vi "SR760FFT_init_measure.vi"(5 "Measure":bool, 7 "Init":bool, 8 "error in":T1, 11 "GPIB address":string="10") -> (0 "error out":T1, 3 "Array":dbl[](array[numeric]))   [LabVIEW 2023]
panel:
  out "trace":dbl[](graph)
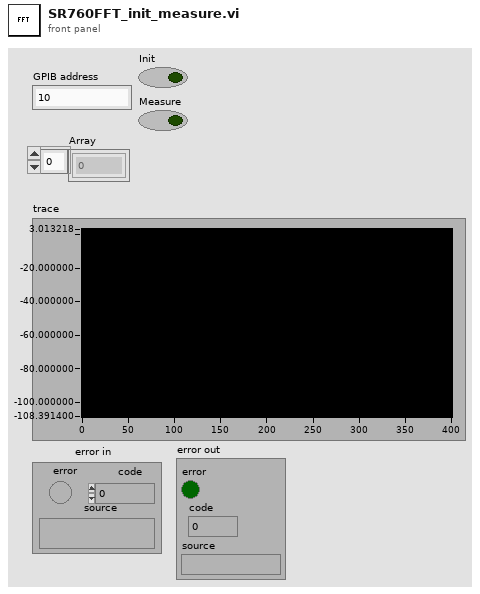
[diagram p1: front panel]
types:
  T1 = cluster{"error":bool, "code":i32, "source":string}
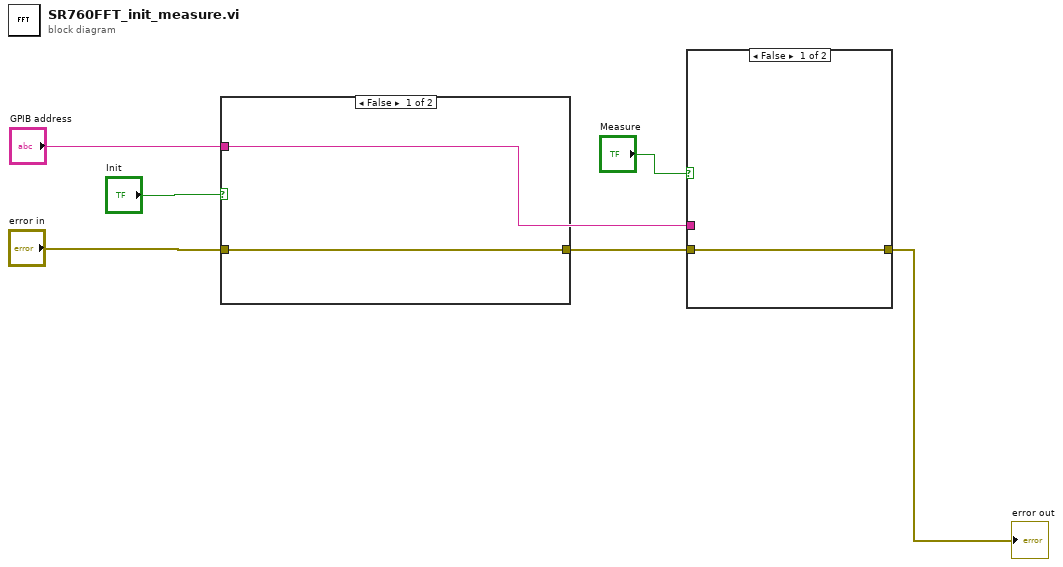
[diagram p0: block diagram]
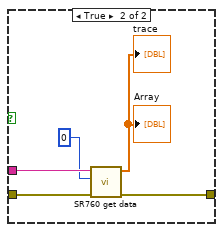
[diagram p2: hidden frame]
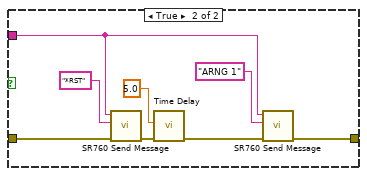
[diagram p3: hidden frame]
diagram:
  n1 = case shown="False" "Init" {
    tunnel: "GPIB address" -> [_ w10]
    tunnel: [w7 w9] -> w5
    tunnel: "error in" -> [w7 w8]
    frame False {
    }
    frame True {
      n2 = call <instrlib>:"SR760 Send Message.vi"("address string"=w10, "write buffer"="*RST", "error in"=w8) -> ("error out"=w13:T1)  [unwired: 4 in, 2 out]
      n3 = call "Time Delay"("error in (no error)"=w13, "Delay Time (s)"=5.0) -> ("error out"=w11:errorcluster)  [unwired: 9 in]
      n4 = call <instrlib>:"SR760 Send Message.vi"("address string"=w10, "write buffer"="ARNG 1", "error in"=w11) -> ("error out"=w9:T1)  [unwired: 4 in, 2 out]
    }
  }
  n5 = case shown="False" "Measure" {
    tunnel: "GPIB address" -> [_ w21]
    tunnel: w5 -> [w16 w19]
    tunnel: [w16 w17] -> w3
    frame False {
    }
    frame True {
      n6 = call "SR760 get data.VI"("error in 2"=w19, "active trace"=i8 0, "GPIB address"=w21) -> ("error out"=w17:T1, "trace"=→"Array" →"trace":dbl[])  [unwired: 7 in]
    }
  }
  "error out" <- w3
